vi "peak - fix phase.vi"(8 "4corners":T1={"z (-pi/2)"=-1.0311345636926572+0.5736824521422934i, "z(inf)"=-0.5200164984937075+1.0975277942502903i, "z (pi/2)"=-1.0311345636926572+0.5736824521422934i, "z center"=-0.5136528600391839+0.580046090596817i, "z(0)"=-0.5200164984937075+1.0975277942502903i, "radius"=-1.0311345636926572}, 10 "correct phase":dbl) -> (0 "4corners out":T1={"z (-pi/2)"=-1.0311345636926572+0.5736824521422934i, "z(inf)"=-0.5200164984937075+1.0975277942502903i, "z (pi/2)"=-1.0311345636926572+0.5736824521422934i, "z center"=-0.5136528600391839+0.580046090596817i, "z(0)"=-0.5200164984937075+1.0975277942502903i, "radius"=-1.0311345636926572})   [LabVIEW 2017]
uses:
  circle corners.ctl
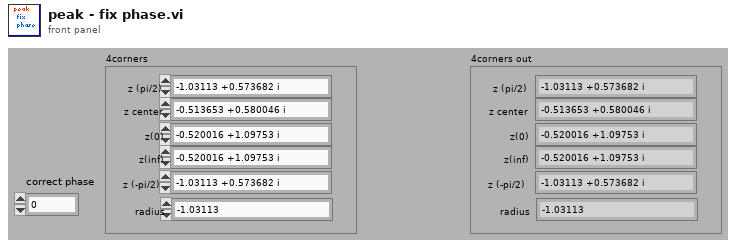
[diagram p1: front panel]
types:
  T1 = typedef "circle corners.ctl" = cluster{"z (-pi/2)":cdb, "z(inf)":cdb, "z (pi/2)":cdb, "z center":cdb, "z(0)":cdb, "radius":dbl}
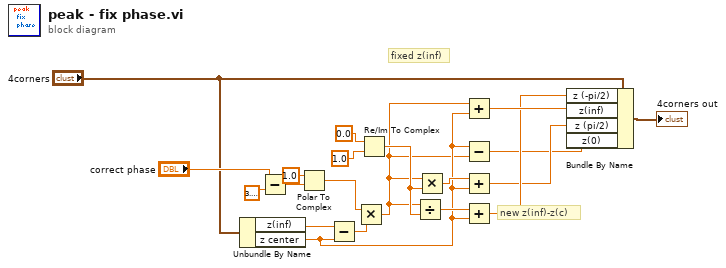
[diagram p0: block diagram]
diagram:
  # "new z(inf)-z(c)"
  # "fixed z(inf)"
  n1 = Unbundle By Name("4corners") -> ("z(inf)"=w16:cdb, "z center"=w2:cdb)
  n2 = Subtract(x="correct phase", y=3.141592653589793) -> (x-y=w14:dbl)
  n3 = Polar To Complex(1:w14, 2:1.0 ("r")) -> (0:w12:cdb)
  n4 = Subtract(x=w16, y=w2) -> (x-y=w15:cdb)
  n5 = Multiply(x=w12, y=w15) -> (x*y=w1:cdb)
  n6 = Re/Im To Complex(1:1.0 ("y"), 2:0.0 ("x")) -> (0:w7:cdb)
  n7 = Divide(x=w1, y=w7) -> (x/y=w8:cdb)
  n8 = Multiply(x=w1, y=w7) -> (x*y=w9:cdb)
  n9 = Add(x=w1, y=w2) -> (x+y=w6:cdb)
  n10 = Subtract(x=w2, y=w1) -> (x-y=w3:cdb)
  n11 = Add(x=w9, y=w2) -> (x+y=w4:cdb)
  n12 = Add(x=w8, y=w2) -> (x+y=w5:cdb)
  n13 = Bundle By Name(cluster="4corners", "z (-pi/2)"=w5, "z(inf)"=w6, "z (pi/2)"=w4, "z(0)"=w3) -> (→"4corners out":T1)
